vi "Scan Setup.vi"(8 "error in (no error)":errorcluster, 11 "Wavelength iHR320 in":refnum<class "Wavelength ActiveX.lvclass">) -> (0 "error out":errorcluster, 3 "Wavelength iHR320 out":refnum<class "Wavelength ActiveX.lvclass">)   [LabVIEW 2017, in "Wavelength ActiveX.lvclass"]
doc: "Configure the Instrument based on the class member fields. This step comes after the user has closed the \"Scan Setup\" window and before the actual scan -- so instruments are configured with the user's specified settings."
uses:
  Wavelength ActiveX.lvclass
  Scanner/Scanner.lvclass
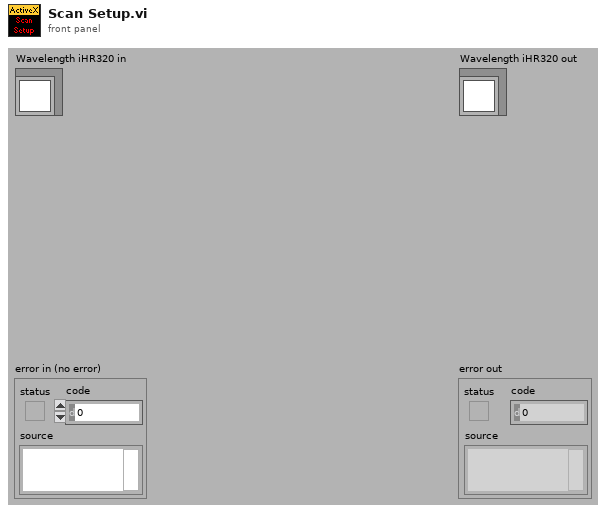
[diagram p1: front panel]
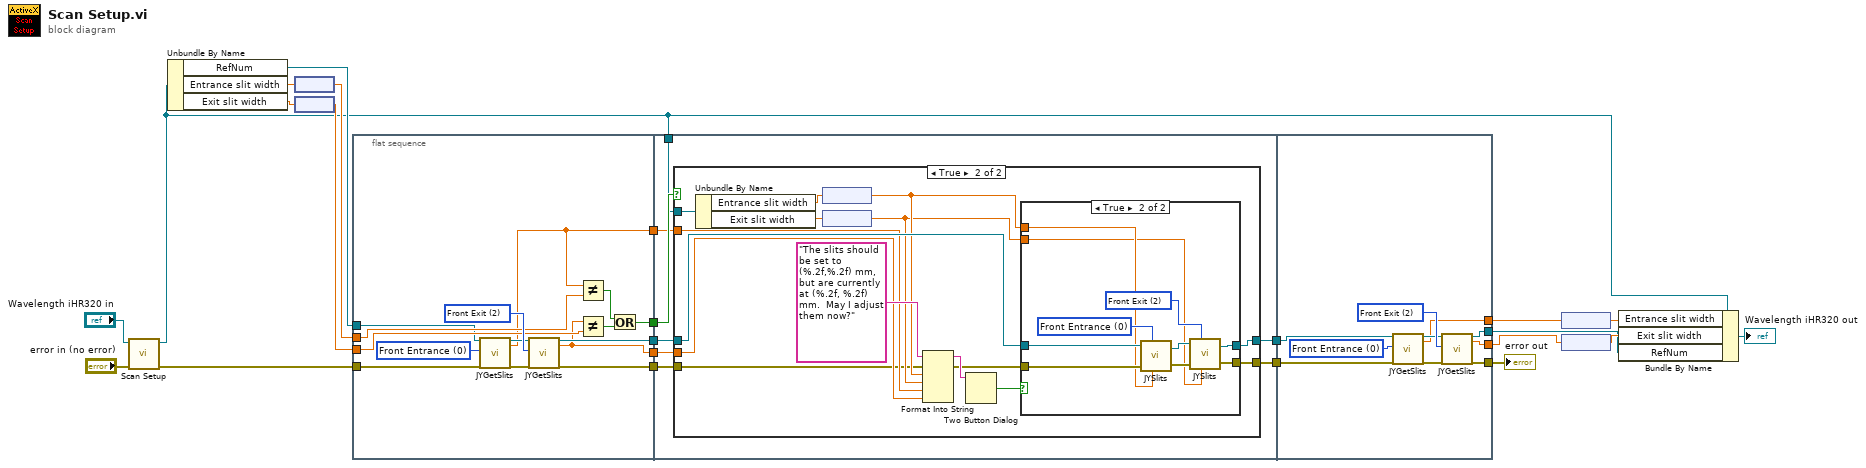
[diagram p0: block diagram]
diagram:
  n1 = call-parent "Scan Setup.vi"("error in (no error)"="error in (no error)", "Scanner in"="Wavelength iHR320 in") -> ("error out"=w5:errorcluster, "Scanner out"=w3:refnum<class "Wavelength ActiveX.lvclass">)  [unwired: 8 in]
  n2 = Unbundle By Name(w3) -> ("RefNum"=w6:refnum<k7>, "Entrance slit width"=w20:dbl[unit], "Exit slit width"=w21:dbl[unit])
  n3 = node(w20) -> (w8:dbl)
  n4 = node(w21) -> (w7:dbl)
  n5 = flat-sequence {
    tunnel: [w30] -> w10
    tunnel: [w27] -> w9
    tunnel: w8 -> [w34]
    tunnel: w7 -> [w33]
    tunnel: w6 -> [w32]
    tunnel: w5 -> [w29]
    tunnel: [w26] -> w4
    tunnel: [w25] -> w2
    tunnel: [w24] -> w1
    tunnel: [w45] -> w18
    tunnel: [w43] -> w17
    tunnel: w10 -> [w46]
    tunnel: w9 -> [w44]
    tunnel: w4 -> [w42]
    tunnel: w3 -> [w41]
    tunnel: w2 -> [w40]
    tunnel: w1 -> [w39]
    tunnel: w18 -> [w83]
    tunnel: w17 -> [w81]
    tunnel: [w79] -> w16
    tunnel: [w78] -> w13
    tunnel: [w77] -> w12
    tunnel: [w76] -> w11
    frame #0 {
      w37 = u16 2 items=["Front Entrance", "Side Entrance", "Front Exit", "Side Exit", "First Intermediate", "Second Intermediate"] ("Slit")
      w38 = u16 0 items=["Front Entrance", "Side Entrance", "Front Exit", "Side Exit", "First Intermediate", "Second Intermediate"] ("Slit")
      n6 = call "JYGetSlits.vi"("MonoRefNum IN"=w32, "Slit"=w38, "error in (no error)"=w29) -> ("MonoRefNum Out"=w31:refnum<k7>, "Slit Width"=w25:dbl, "error out"=w28:errorcluster)  [unwired: 13 in, 1 out]
      n7 = call "JYGetSlits.vi"("MonoRefNum IN"=w31, "Slit"=w37, "error in (no error)"=w28) -> ("MonoRefNum Out"=w30:refnum<k7>, "Slit Width"=w24:dbl, "error out"=w27:errorcluster)  [unwired: 13 in, 1 out]
      n8 = Not Equal?(x=w25, y=w34) -> (x != y?=w35:bool)
      n9 = Not Equal?(x=w24, y=w33) -> (x != y?=w36:bool)
      n10 = Or(x=w35, y=w36) -> (x .or. y?=w26:bool)
    }
    frame #1 {
      n11 = case shown="True" w42 {
        tunnel: w46 -> [w47 w63]
        tunnel: [w47 w62] -> w45
        tunnel: w44 -> [w48 w50]
        tunnel: [w48 w61] -> w43
        tunnel: w41 -> [_ w58]
        tunnel: w40 -> [_ w57]
        tunnel: w39 -> [_ w56]
        frame False {
        }
        frame True {
          n12 = Unbundle By Name(w58) -> ("Entrance slit width"=w54:dbl[unit], "Exit slit width"=w52:dbl[unit])
          n13 = node(w54) -> (w53:dbl)
          n14 = node(w52) -> (w51:dbl)
          n15 = Format Into String(initial string="The slits should be set to (%.2f,%.2f) mm, but are currently at (%.2f, %.2f) mm.  May I adjust them now?", error in=w50, w53, w51, w57, w56) -> (resulting string=w59:string, error out=w49:errorcluster)  [unwired: 1 in]
          n16 = Two Button Dialog(message=w59) -> (T button?=w55:bool)  [unwired: 2 out]
          n17 = case shown="True" w55 {
            tunnel: w63 -> [w65 w72]
            tunnel: [w65 w71] -> w62
            tunnel: w49 -> [w64 w70]
            tunnel: [w64 w68] -> w61
            tunnel: w53 -> [_ w67]
            tunnel: w51 -> [_ w66]
            frame False {
            }
            frame True {
              w75 = u16 2 items=["Front Entrance", "Side Entrance", "Front Exit", "Side Exit", "First Intermediate", "Second Intermediate"] ("Slit")
              w73 = u16 0 items=["Front Entrance", "Side Entrance", "Front Exit", "Side Exit", "First Intermediate", "Second Intermediate"] ("Slit")
              n18 = call "JYSlits.vi"("JYMONOLib.IJYMonoReqd In"=w72, "Slit"=w73, "error in (no error)"=w70, "Slit Width"=w67) -> ("JYMONOLib.IJYMonoReqd Out"=w74:refnum<k7>, "error out"=w69:errorcluster)  [unwired: 1 in]
              n19 = call "JYSlits.vi"("JYMONOLib.IJYMonoReqd In"=w74, "Slit"=w75, "error in (no error)"=w69, "Slit Width"=w66) -> ("JYMONOLib.IJYMonoReqd Out"=w71:refnum<k7>, "error out"=w68:errorcluster)  [unwired: 1 in]
            }
          }
        }
      }
    }
    frame #2 {
      w84 = u16 2 items=["Front Entrance", "Side Entrance", "Front Exit", "Side Exit", "First Intermediate", "Second Intermediate"] ("Slit")
      w85 = u16 0 items=["Front Entrance", "Side Entrance", "Front Exit", "Side Exit", "First Intermediate", "Second Intermediate"] ("Slit")
      n20 = call "JYGetSlits.vi"("MonoRefNum IN"=w83, "Slit"=w85, "error in (no error)"=w81) -> ("MonoRefNum Out"=w82:refnum<k7>, "Slit Width"=w78:dbl, "error out"=w80:errorcluster)  [unwired: 13 in, 1 out]
      n21 = call "JYGetSlits.vi"("MonoRefNum IN"=w82, "Slit"=w84, "error in (no error)"=w80) -> ("MonoRefNum Out"=w76:refnum<k7>, "Slit Width"=w77:dbl, "error out"=w79:errorcluster)  [unwired: 13 in, 1 out]
    }
  }
  n22 = node(w13) -> (w14:dbl[unit])
  n23 = node(w12) -> (w15:dbl[unit])
  n24 = Bundle By Name(cluster=w3, "Entrance slit width"=w14, "Exit slit width"=w15, "RefNum"=w11) -> (→"Wavelength iHR320 out":refnum<class "Wavelength ActiveX.lvclass">)
  "error out" <- w16
